vi "lv_mysql_conn_send_data_packet.vi"(6 "timeout ms (5000)":i32=5000, 8 "error in":errorcluster, 9 "TCP/IP Data":u8[](array[numeric]), 10 "Packet #":u8, 11 "connection ID":refnum<k5>) -> (0 "error out":errorcluster, 3 "connection ID out":refnum<k5>)   [LabVIEW 2010]
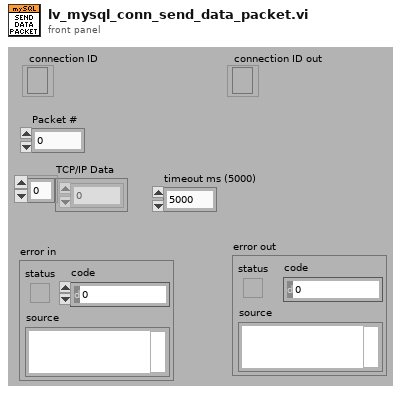
[diagram p1: front panel]
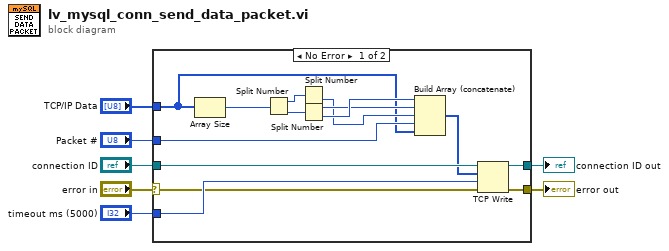
[diagram p0: block diagram]
diagram:
  n1 = case shown="No Error" "error in" {
    selector: "error in" -> [w8 w23]
    tunnel: "timeout ms (5000)" -> [w21 _]
    tunnel: "connection ID" -> [w20 w22]
    tunnel: [w19 w23] -> w5
    tunnel: [w18 w22] -> w4
    tunnel: "Packet #" -> [w11 _]
    tunnel: "TCP/IP Data" -> [w10 _]
    frame No Error {
      n2 = Array Size(array=w10) -> (size(s)=w9:i32)
      n3 = Split Number(x=w9) -> (hi(x)=w17:u16, lo(x)=w16:u16)
      n4 = Split Number(x=w17) -> (lo(x)=w13:u8)  [unwired: 1 out]
      n5 = Split Number(x=w16) -> (hi(x)=w14:u8, lo(x)=w15:u8)
      n6 = Build Array (concatenate)(w15, w14, w13, w11, w10) -> (w12:u8[])
      n7 = TCP Write(connection ID=w20, data in=w12, error in (no error)=w8, 9:w21) -> (connection ID out=w18:refnum<k5>, error out=w19:errorcluster)  [unwired: 1 out]
    }
    frame Error {
    }
  }
  "connection ID out" <- w4
  "error out" <- w5
